vi "Draw Geometric Matches Position .vi"(10 "Matches (pixel)":T1[](array[typedef]) {"Correlation Score" format="%.2f"; "Target Template Curve Score" format="%.2f"; "Template Target Curve Score" format="%.2f"; "Bounding Box"."y" format="%.2f"; "Bounding Box"."x" format="%.2f"; "Position"."y" format="%.2f"; "Position"."x" format="%.2f"; "Score" format="%.2f"; "Scale" format="%.2f"; "Angle" format="%.2f"; "Occlusion %" format="%.2f"}, 11 "Image":T2) -> (3 "Image Out":T2)   [LabVIEW 2019]
uses:
  <vilib>/vision/Image Controls.llb/IMAQ Image.ctl
  <vilib>/vision/Pattern Matching.llb/IMAQ GM Match Report.ctl
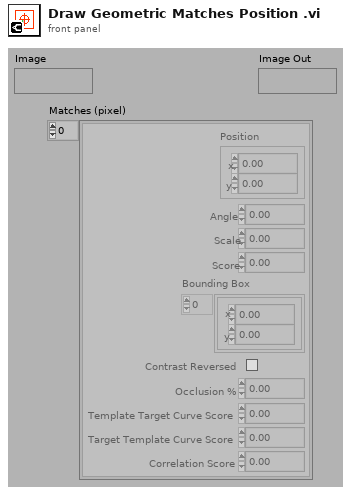
[diagram p1: front panel]
types:
  T1 = typedef "IMAQ GM Match Report.ctl" = cluster{"Position":cluster{"x":sgl, "y":sgl}, "Angle":sgl, "Scale":sgl, "Score":sgl, "Bounding Box":cluster{"x":sgl, "y":sgl}[], "Contrast Reversed":bool, "Occlusion %":sgl, "Template Target Curve Score":sgl, "Target Template Curve Score":sgl, "Correlation Score":sgl}
  T2 = typedef "IMAQ Image.ctl" = refnum<image>
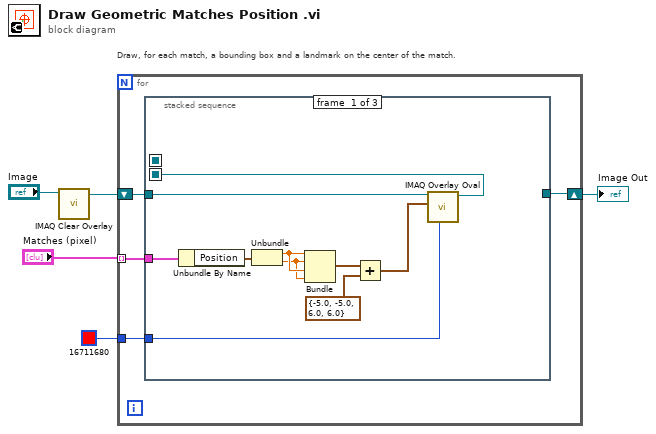
[diagram p0: block diagram]
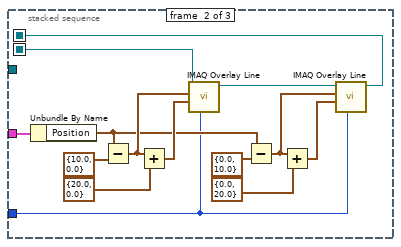
[diagram p2: hidden frame]
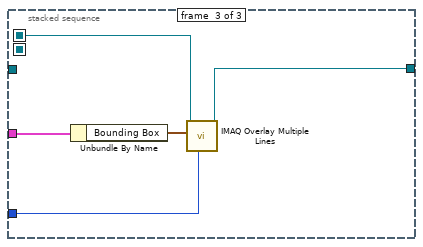
[diagram p3: hidden frame]
diagram:
  # "Draw, for each match, a bounding box and a landmark on the center of the match."
  n1 = call "IMAQ Clear Overlay"("Image"="Image") -> ("Image Out"=w3:T2)  [unwired: 2 in, 8 out]
  n2 = for {
    shift-right: [w6] -> w5
    shift-left: w3 -> [w8]
    tunnel: "Matches (pixel)" -> [w9] mode=indexing
    tunnel: u32 16711680 ("color(black)") -> [w7]
    n3 = stacked-sequence {
      seq-local: [w17 _ _] -> [_ w31 _]
      seq-local: [_ w21 _] -> [_ _ w37]
      tunnel: w9 -> [w19 w33 w38]
      tunnel: w8 -> [w18 _ _]
      tunnel: w7 -> [w16 w22 w35]
      tunnel: [_ _ w36] -> w6
      frame #0 {
        n4 = Unbundle By Name(w19) -> ("Position"=w15:cluster{"x":sgl, "y":sgl})
        n5 = Unbundle(w15) -> ("x"=w14:sgl, "y"=w13:sgl)
        n6 = Bundle("x"=w14, "y"=w13, "x"=w14, "y"=w13) -> (w12:cluster{"x":sgl, "y":sgl, "x":sgl, "y":sgl})  [unwired: 1 out]
        n7 = Add(x=w12, y=cluster{"y":sgl, "x":sgl, "y":sgl, "x":sgl} {"y"=-5.0, "x"=-5.0, "y"=6.0, "x"=6.0}) -> (x+y=w10:cluster{sgl, sgl, sgl, sgl})
        n8 = call "IMAQ Overlay Oval"("Color"=w16, "Bounding Rectangle"=w10, "Image"=w18) -> ("Image Out"=w17:T2)  [unwired: 3 in, 5 out]
      }
      frame #1 {
        n9 = Unbundle By Name(w33) -> ("Position"=w24:cluster{"x":sgl, "y":sgl})
        n10 = Subtract(x=w24, y=cluster{"x":sgl, "y":sgl} {"x"=10.0, "y"=0.0}) -> (x-y=w30:cluster{"x":sgl, "y":sgl})
        n11 = Add(x=w30, y=cluster{"x":sgl, "y":sgl} {"x"=20.0, "y"=0.0}) -> (x+y=w28:cluster{"x":sgl, "y":sgl})
        n12 = call "IMAQ Overlay Line"("Color"=w22, "End Point"=w28, "Start Point"=w30, "Image"=w31) -> ("Image Out"=w20:T2)  [unwired: 2 in, 5 out]
        n13 = Subtract(x=w24, y=cluster{"x":sgl, "y":sgl} {"x"=0.0, "y"=10.0}) -> (x-y=w26:cluster{"x":sgl, "y":sgl})
        n14 = Add(x=w26, y=cluster{"x":sgl, "y":sgl} {"x"=0.0, "y"=20.0}) -> (x+y=w27:cluster{"x":sgl, "y":sgl})
        n15 = call "IMAQ Overlay Line"("Color"=w22, "End Point"=w27, "Start Point"=w26, "Image"=w20) -> ("Image Out"=w21:T2)  [unwired: 2 in, 5 out]
      }
      frame #2 {
        n16 = Unbundle By Name(w38) -> ("Bounding Box"=w34:cluster{"x":sgl, "y":sgl}[])
        n17 = call "IMAQ Overlay Multiple Lines"("Color"=w35, "Line End Points"=w34, "Image"=w37) -> ("Image Out"=w36:T2)  [unwired: 3 in, 5 out]
      }
    }
  }
  "Image Out" <- w5
